vi "Telemetry Session Assurance.vi"(8 "error in":errorcluster, 11 "MICS Dongle Address":refnum<visa-resource-name>="COM11") -> (0 "error out":errorcluster, 3 "MICS Dongle Address dup":refnum<visa-resource-name>)   [LabVIEW 2020]
uses:
  Typedef Command List.ctl
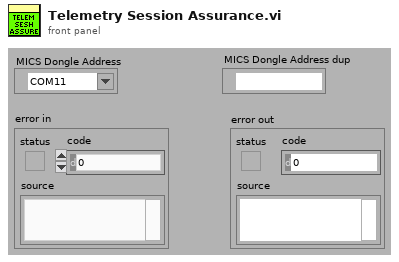
[diagram p1: front panel]
types:
  T1 = typedef "Typedef Command List.ctl" = enum16{"Get xPG Status", "xPG Stimulation", "Select Program", "Increment Program Amplitude", "Decrement Program Amplitude", "Get PoP Constants", "Get PPC Constants", "Get Program Names", "Set Pulse Amplitude", "Increment Pulse Amplitude", "Decrement Pulse Amplitude", "Get Pulse Widths", "Set Pulse Widths", "Increment Pulse Width", "Decrement Pulse Width", "Get Program Frequency", "Set Program Frequency", "Increment Program Frequency", "Decrement Program Frequency", "Inject Event", "Charging Control", "Get xPG Identity", "Set xPG Identity", "Restore Program Defaults", "Get Program Definition", "Set Program Definition", "Get Program Constants", "Set Program Constants", "Get Configurable Device Parameters", "Set Configurable Device Parameters", "Get Pulse Constants", "Set Pulse Constants", "Get Lead Limits", "Set Lead Limits", "Get Channel Calibrations", "Set Channel Calibrations", "<reserved 2>", "<reserved 3>", "<reserved 4>", "<reserved 5>", "<reserved 6>", "<reserved 7>", "Get Stim Asic HV Calibrations", "Set Stim Asic HV Calibrations", "<reserved 8>", "<reserved 9>", "Get CP Data", "Set CP Data", "Clear Log", "Read Log", "Append Log", "Get Patient Program Runtime", "Set Patient Program Runtime", "Impedance Measurement", "Enter Storage Mode", "Echo Short", "Echo Long", "Get General Calibration", "Set General Calibration", "Get Trim List", "Set Trim List", "Get Counter", "Set Counter", "Get Test Stimulation", "Set Test Stimulation", "Get Titration Stimulation", "Set Titration Stimulation", "Get Ramp Time", "Set Ramp Time", "Get VBAT", "Set Software Description Block", "Get Software Description Block", "Write Memory", "Read Memory", "Reset xPG", "Erase Flash Block", "Write Vectors", "Read Vectors", "Diagnostic Data", "Set Background Impedance", "Get Background Impedence ", "Set Test Waveform", "Calibrate Channel", "Get Log Range", "Reserved 0x55", "Reserved 0x56", "MICS Options", "Pair PPC", "Pair POP", "Stop Bootloader", "Tune MICS", "MICS Diagnostics", "Undefined"}
  T2 = cluster{"Command":T1, "Function":enum16{"Open Session", "Close Session", "Downlink Only", "Uplink Only", "Transceive (DN -> UP)"}, "MICS_ID":u32, "EXID":u32, "Use Local":bool, "Transceive Delay mS":dbl, "CP_DATA IN":u8[], "Parameters":string}
  T3 = cluster{"Response Token":string, "Response Code":string, "bChecksum Valid":bool, "tChecksum Valid":bool, "CP_DATA OUT":u8[], "Data":string}
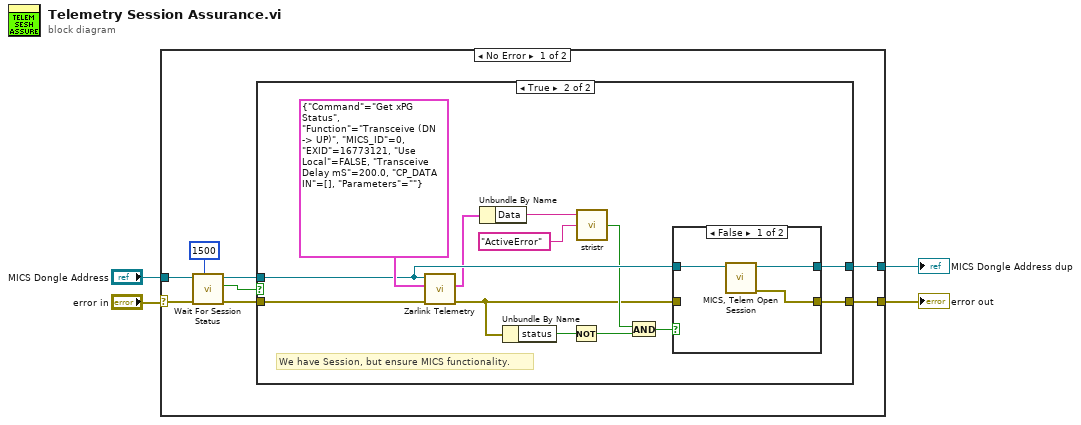
[diagram p0: block diagram]
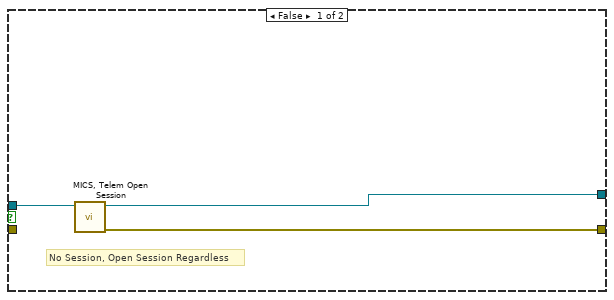
[diagram p2: hidden frame]
diagram:
  n1 = case shown="No Error" "error in" {
    selector: "error in" -> [w12 w35]
    tunnel: [w8 w35] -> w2
    tunnel: "MICS Dongle Address" -> [w7 w34]
    tunnel: [w6 w34] -> w1
    frame No Error {
      n2 = call "Wait For Session Status.vi"("Timeout (3000 ms)"=u32 1500, "error in (no error)"=w12, "VISA Resource Name"=w7) -> ("error out"=w9:errorcluster, "IN_SESSION"=w11:bool, "dup VISA Resource Name"=w10:refnum<visa-resource-name>)  [unwired: 5 in, 1 out]
      n3 = case shown="True" w11 {
        tunnel: w9 -> [_ w28]
        tunnel: w10 -> [w15 w26]
        tunnel: [w14 w17] -> w8
        tunnel: [w13 w16] -> w6
        frame False {
          # "No Session, Open Session Regardless"
          n4 = call "MICS, Telem Open Session.vi"("VISA resource"=w15) -> ("error out"=w14:errorcluster, "VISA resource dup"=w13:refnum<visa-resource-name>)  [unwired: 8 in, 1 out]
        }
        frame True {
          # "We have Session, but ensure MICS functionality."
          n5 = call "Zarlink Telemetry.vi"("error in (no error)"=w28, "Input"=T2 {"Command"=enum."Get xPG Status", "Function"=enum."Transceive (DN -> UP)", "MICS_ID"=0, "EXID"=16773121, "Use Local"=FALSE, "Transceive Delay mS"=200.0, "CP_DATA IN"=[], "Parameters"=""}, "MICS Dongle Address"=w26) -> ("error out"=w18:errorcluster, "Output"=w23:T3)  [unwired: 6 in, 1 out]
          n6 = Unbundle By Name(w23) -> ("Data"=w24:string)
          n7 = Unbundle By Name(w18) -> ("status"=w21:bool)
          n8 = Not(x=w21) -> (.not. x?=w19:bool)
          n9 = call "stristr.vi"("Substring"="ActiveError" ("regular expression"), "Input String"=w24) -> ("found"=w20:bool)  [unwired: 1 in, 2 out]
          n10 = And(x=w20, y=w19) -> (x .and. y?=w22:bool)
          n11 = case shown="False" w22 {
            tunnel: w26 -> [w31 w32]
            tunnel: w18 -> [_ w33]
            tunnel: [w30 w33] -> w17
            tunnel: [w29 w32] -> w16
            frame False {
              n12 = call "MICS, Telem Open Session.vi"("VISA resource"=w31) -> ("error out"=w30:errorcluster, "VISA resource dup"=w29:refnum<visa-resource-name>)  [unwired: 8 in, 1 out]
            }
            frame True {
            }
          }
        }
      }
    }
    frame Error {
    }
  }
  "error out" <- w2
  "MICS Dongle Address dup" <- w1
